vi "Create Error.vi"(7 "Call Chain (F)":bool, 9 "MultiErrors in":refnum<class "MultiErrors.lvclass">, 10 "Message":string, 11 "Code":i32=1) -> (1 "MultiErrors out":refnum<class "MultiErrors.lvclass">)   [LabVIEW 2020, in "VolatusErrorUtilities.lvlib" / "MultiErrors.lvclass"]
uses:
  MultiErrors.lvclass
  MultiError.ctl
  MultiErrors.lvclass/MultiErrors.ctl
  VolatusErrorUtilities.lvlib
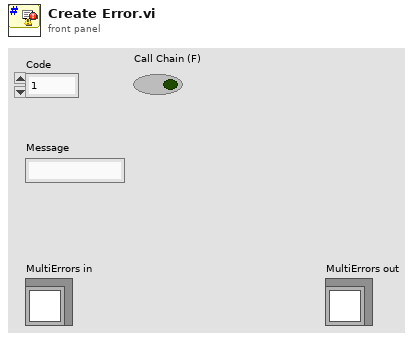
[diagram p1: front panel]
types:
  T1 = typedef "VolatusErrorUtilities.lvlib/MultiError.ctl" = cluster{"Context":string[], "Message":string, "Code":i32, "Call Chain":string[]}
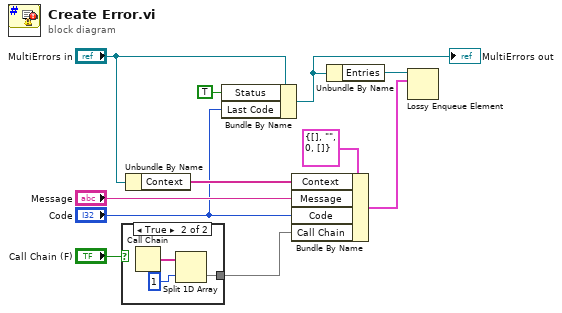
[diagram p0: block diagram]
diagram:
  n1 = case shown="True" "Call Chain (F)" {
    tunnel: [_ w12] -> w7
    frame False {
    }
    frame True {
      n2 = Call Chain() -> (call chain=w14:string[])
      n3 = Split 1D Array(array=w14, index=1) -> (second subarray=w12:string[])  [unwired: 1 out]
    }
  }
  n4 = Unbundle By Name("MultiErrors in") -> ("Context"=w10:string[])
  n5 = Bundle By Name(cluster="MultiErrors in", "Status"=TRUE, "Last Code"="Code") -> (w3:refnum<class "MultiErrors.lvclass">)
  "MultiErrors out" <- w3
  n6 = Bundle By Name(cluster=T1 {"Context"=[], "Message"="", "Code"=0, "Call Chain"=[]} ("MultiError Entry"), "Context"=w10, "Message"="Message", "Code"="Code", "Call Chain"=w7) -> (w5:T1)
  n7 = Unbundle By Name(w3) -> ("Entries"=w6:refnum<queue>)
  n8 = Lossy Enqueue Element(queue=w6, element=w5) -> ()  [unwired: 1 in, 4 out]
